vi "CTRE_PigeonIMU_Open_CAN.vi"(8 "error in":errorcluster, 10 "Device Number":u8) -> (0 "error out":errorcluster, 3 "PigeonIMUDevRef":T1={"DeviceStatus"={"status"=FALSE, "code"=0, "source"=""}, "Device Number"=0, "Type"=352321536, "Device ID"=0, "Handle"=0, "UsageFrame"=0, "Library Path"=path ""} {"Type" items=["CAN"=352321536, "TalonSRX"=33554432]})   [LabVIEW 2016]
doc: "Opens a Pigeon IMU Device Reference using a CAN ID."
uses:
  <vilib>/Rock Robotics/WPI/ThirdParty/Sensors/Pigeon IMU/CTRE_PigeonIMU_DeviceRef.ctl
  <vilib>/Rock Robotics/WPI/ThirdParty/Sensors/Pigeon IMU/CTRE_PigeonIMU_ConnectionType.ctl
  <vilib>/Rock Robotics/WPI/ThirdParty/Sensors/Pigeon IMU/CTRE_PigeonIMU_UsageTypes.ctl
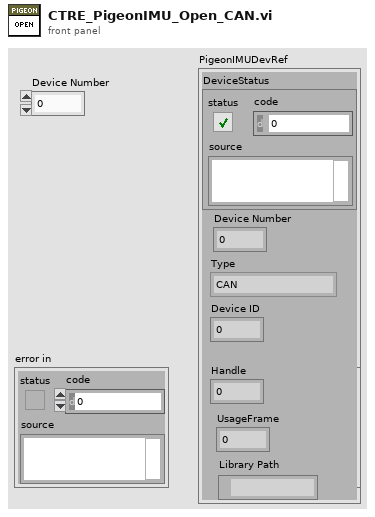
[diagram p1: front panel]
types:
  T1 = typedef "CTRE_PigeonIMU_DeviceRef.ctl" = cluster{"DeviceStatus":errorcluster, "Device Number":u8, "Type":T2, "Device ID":u32, "Handle":u64, "UsageFrame":u32, "Library Path":path}
  T2 = typedef "CTRE_PigeonIMU_ConnectionType.ctl" = u32
  T3 = typedef "CTRE_PigeonIMU_UsageTypes.ctl" = u32
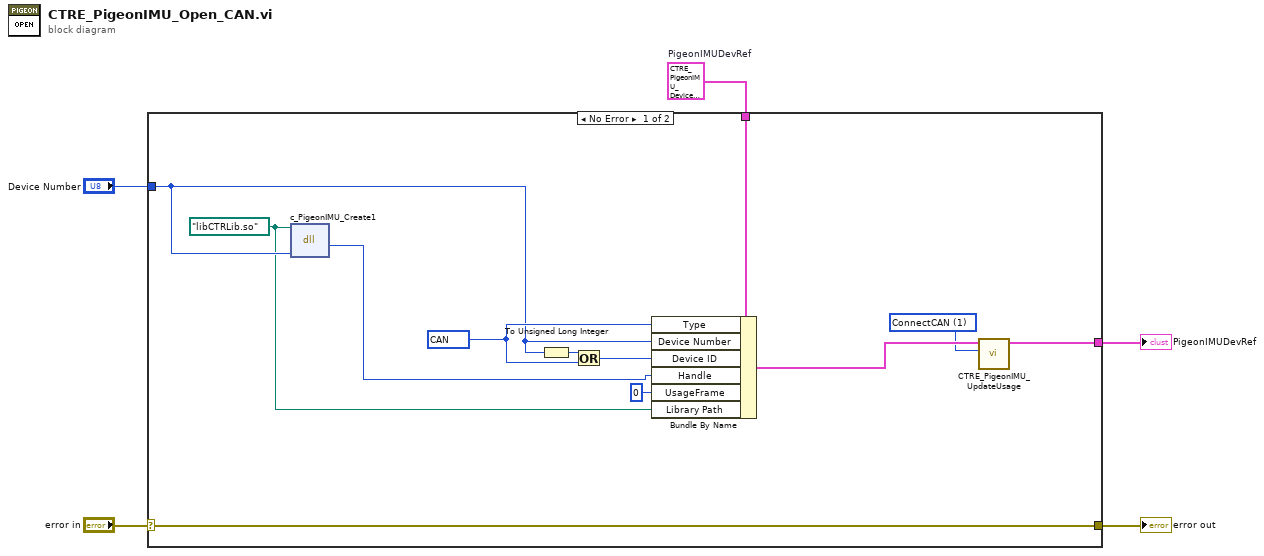
[diagram p0: block diagram]
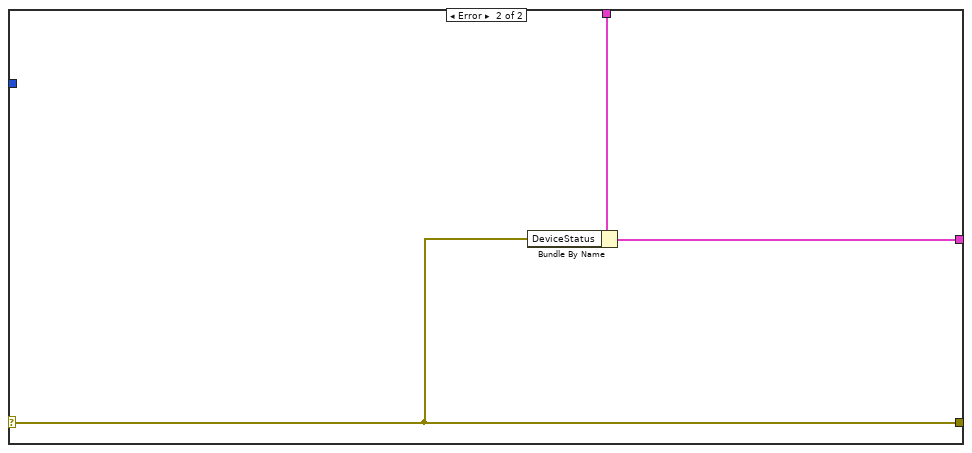
[diagram p2: hidden frame]
diagram:
  w3 = T1 {"DeviceStatus"={"status"=FALSE, "code"=0, "source"=""}, "Device Number"=0, "Type"=352321536, "Device ID"=0, "Handle"=0, "UsageFrame"=0, "Library Path"=path ""}  # PigeonIMUDevRef
  n1 = case shown="No Error" "error in" {
    selector: "error in" -> [w17 w19]
    tunnel: [w17 w19] -> w4
    tunnel: w3 -> [w16 w20]
    tunnel: [w10 w18] -> w2
    tunnel: "Device Number" -> [w9 _]
    frame No Error {
      w8 = path "libCTRLib.so" ("path in")
      w11 = T3 1 items=["Defaul"=0, "ConnectCAN"=1, "ConnectTalonSRX"=2, "GetCompass"=134217728, "GetYPR"=268435456, "GetFused"=536870912, "GetAccel"=1073741824, "TempComp"=2147483648] ("Usage")
      w13 = T2 352321536 items=["CAN"=352321536, "TalonSRX"=33554432] ("Connection Type")
      n2 = dll-call lib="?" fn="c_PigeonIMU_Create1"(path in=w8, "deviceNumber"=w9) -> ("return type"=w7:u64)  [unwired: 3 in, 2 out]
      n3 = To Unsigned Long Integer(number=w9) -> (unsigned 32bit integer=w15:u32)
      n4 = Or(x=w15, y=w13) -> (x .or. y?=w14:T2)
      n5 = Bundle By Name(cluster=w16, "Type"=w13, "Device Number"=w9, "Device ID"=w14, "Handle"=w7, "UsageFrame"=u32 0, "Library Path"=w8) -> (w12:T1)
      n6 = call <vilib>:"CTRE_PigeonIMU_UpdateUsage.vi"("Usage"=w11, "PigeonIMUDevRef"=w12) -> ("PigeonIMUDevRef"=w10:T1)  [unwired: 9 in]
    }
    frame Error {
      n7 = Bundle By Name(cluster=w20, "DeviceStatus"=w19) -> (w18:T1)
    }
  }
  "error out" <- w4
  "PigeonIMUDevRef" <- w2
